vi "Or.vi"(2 "B":bool, 3 "A":bool) -> (0 "Output":bool)   [LabVIEW 2020, in "Hack.lvlib"]
uses:
  Hack.lvlib
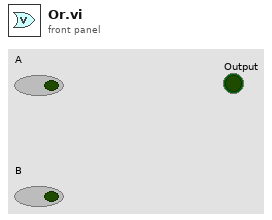
[diagram p1: front panel]
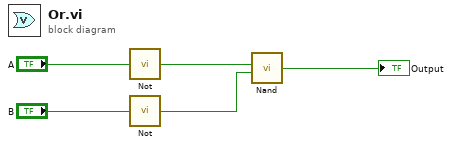
[diagram p0: block diagram]
diagram:
  n1 = call "Not.vi"("Input"="A") -> ("Output"=w3:bool)
  n2 = call "Not.vi"("Input"="B") -> ("Output"=w2:bool)
  n3 = call "Nand.vi"("B"=w2, "A"=w3) -> ("Output"=→"Output":bool)  [unwired: 2 in]
